vi "PointInRect.vi"(8 "错误输入":errorcluster, 10 "point":cluster{"x":dbl, "y":dbl} caption="点" {"y" format="%.2f"; "x" format="%.2f"}, 11 "rect":T1 caption="矩形") -> (0 "错误输出":errorcluster, 2 "pt in rect":bool caption="矩形中的点")   [LabVIEW 2011, in "Rect Tools.lvlib"]
uses:
  Rect Tools.lvlib
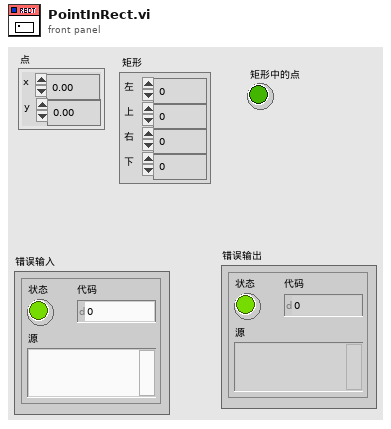
[diagram p1: front panel]
types:
  T1 = cluster{"left":i16, "top":i16, "right":i16, "bottom":i16}
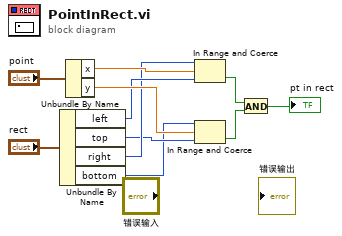
[diagram p0: block diagram]
diagram:
  n1 = Unbundle By Name("rect") -> ("left"=w7:i16, "top"=w5:i16, "right"=w6:i16, "bottom"=w4:i16)
  n2 = Unbundle By Name("point") -> ("x"=w9:dbl, "y"=w8:dbl)
  n3 = In Range and Coerce(upper limit=w6, x=w9, lower limit=w7) -> (In Range?=w3:bool)  [unwired: 1 out]
  n4 = In Range and Coerce(upper limit=w4, x=w8, lower limit=w5) -> (In Range?=w2:bool)  [unwired: 1 out]
  n5 = And(x=w3, y=w2) -> (x .and. y?=→"pt in rect":bool)
